vi "Plotter_Continuous_Receiver.vi"(8 "error in (no error)":errorcluster, 11 "Global Variables":T1) -> ()   [LabVIEW 2017]
uses:
  Controls/Plotter_Globals.ctl
  Classes/ADCP.lvclass
  Controls/Plotter_Queues.ctl
  Controls/Plotter_Queue_Command_and_Data.ctl
  Controls/Plotter_Commands.ctl
  <vilib>/Instr/_visa.llb/VISA Flush IO Buffer Mask.ctl
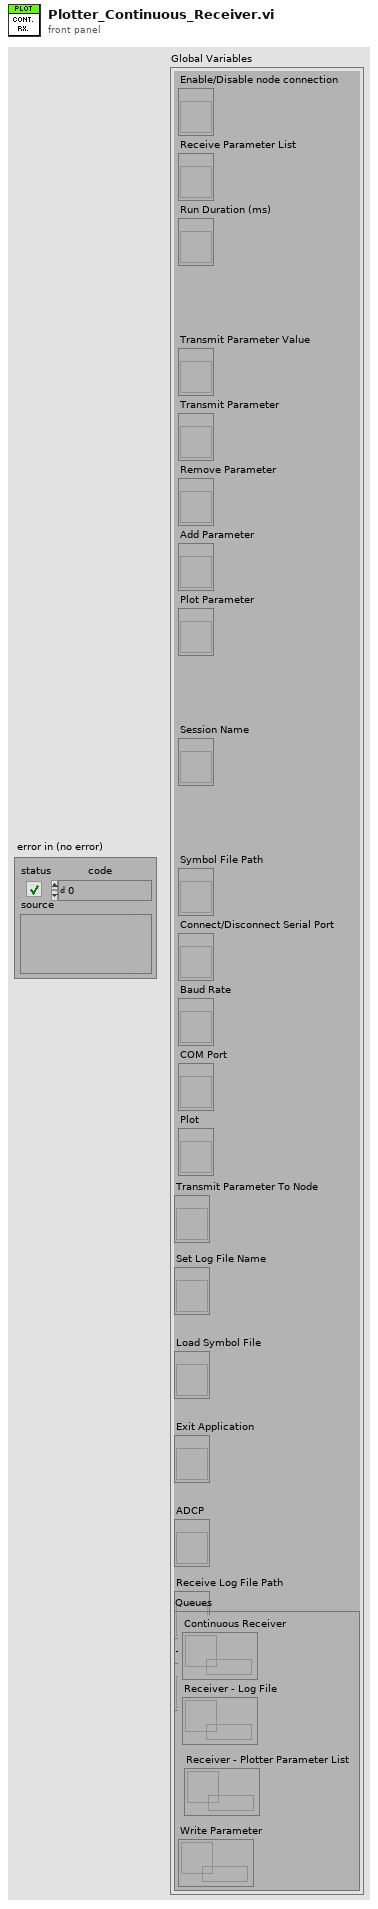
[diagram p1: front panel]
types:
  T1 = typedef "Plotter_Globals.ctl" = cluster{"Enable/Disable node connection":refnum<vi>, "Receive Parameter List":refnum<vi>, "Run Duration (ms)":refnum<vi>, "Transmit Parameter Value":refnum<vi>, "Transmit Parameter":refnum<vi>, "Remove Parameter":refnum<vi>, "Add Parameter":refnum<vi>, "Plot Parameter":refnum<vi>, "Session Name":refnum<vi>, "Symbol File Path":refnum<vi>, "Connect/Disconnect Serial Port":refnum<vi>, "Baud Rate":refnum<vi>, "COM Port":refnum<vi>, "Plot":refnum<vi>, "Transmit Parameter To Node":refnum<vi>, "Set Log File Name":refnum<vi>, "Load Symbol File":refnum<vi>, "Exit Application":refnum<vi>, "ADCP":refnum<vi>, "Transmit Log File Path":refnum<vi>, "Receive Log File Path":refnum<vi>, "Queues":T2}
  T2 = typedef "Plotter_Queues.ctl" = cluster{"Continuous Receiver":refnum<queue>, "Receiver - Log File":refnum<queue>, "Receiver - Plotter Parameter List":refnum<queue>, "Write Parameter":refnum<queue>}
  T3 = typedef "Plotter_Commands.ctl" = enum16{"Idle", "Cont_RX_Open_Node", "Cont_RX_Flush_Serial_Port", "Cont_Rx_Log_Write", "Plot_Update", "Exit"}
  T4 = typedef "Plotter_Queue_Command_and_Data.ctl" = cluster{"Commands":T3, "Data":variant}
  T5 = typedef "VISA Flush IO Buffer Mask.ctl" = u16
  T6 = typedef "ADCP.lvclass/ADCP_Packet_Info.ctl" = cluster{"Priority":enum16{"LOW", "HIGH"}, "Type":enum16{"Data", "Connection Management", "Remote Request", "Error and status", "INVALID"}, "Node ID":i32, "Frame ID":i32, "Checksum valid ?":bool, "Current time (ms)":u32}
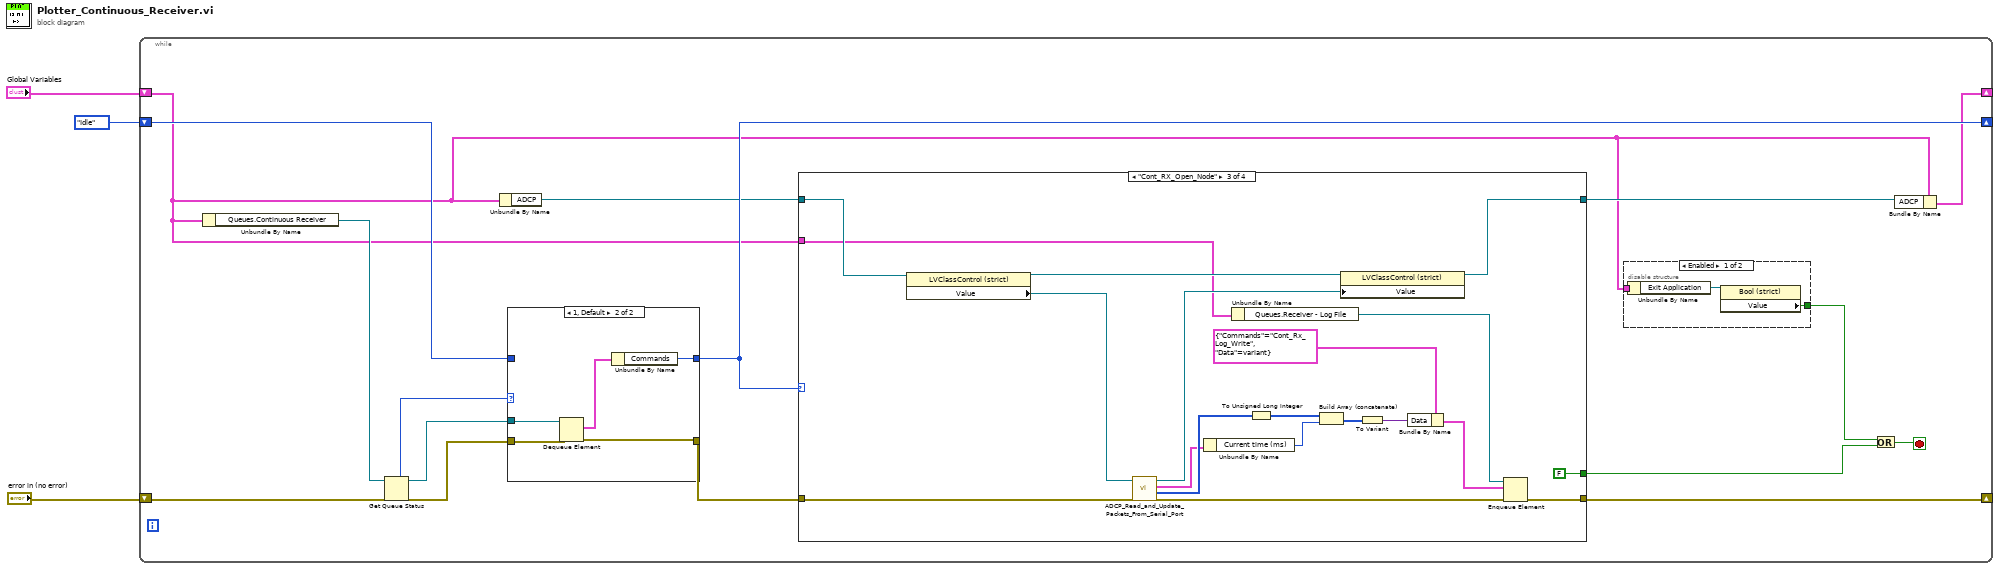
[diagram p0: block diagram]
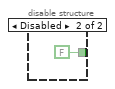
[diagram p2: hidden frame]
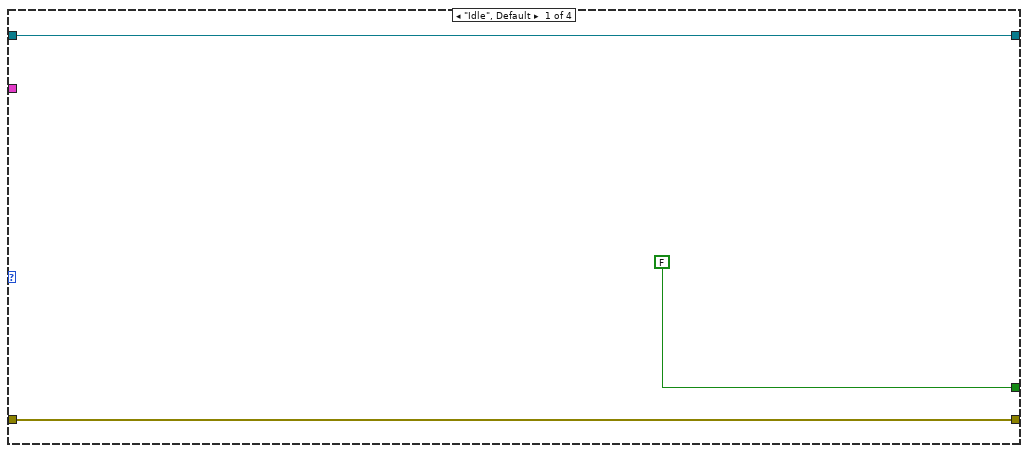
[diagram p3: hidden frame]
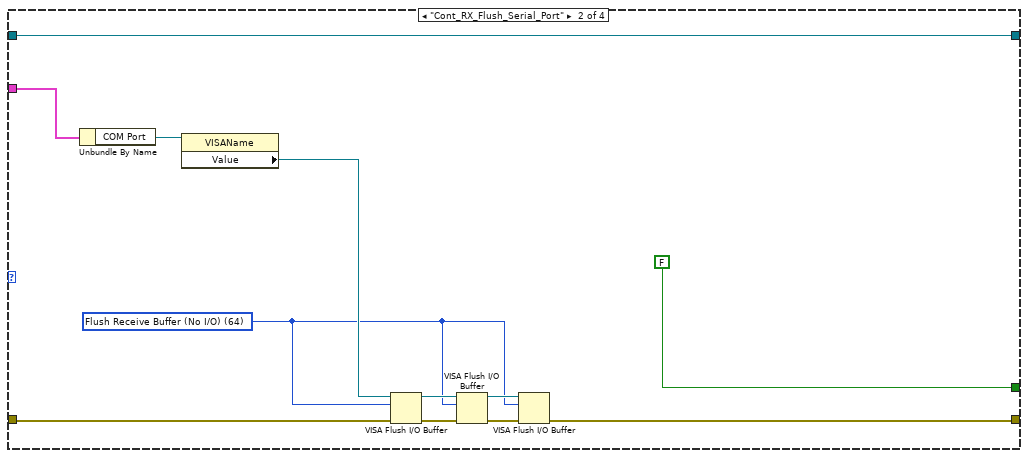
[diagram p4: hidden frame]
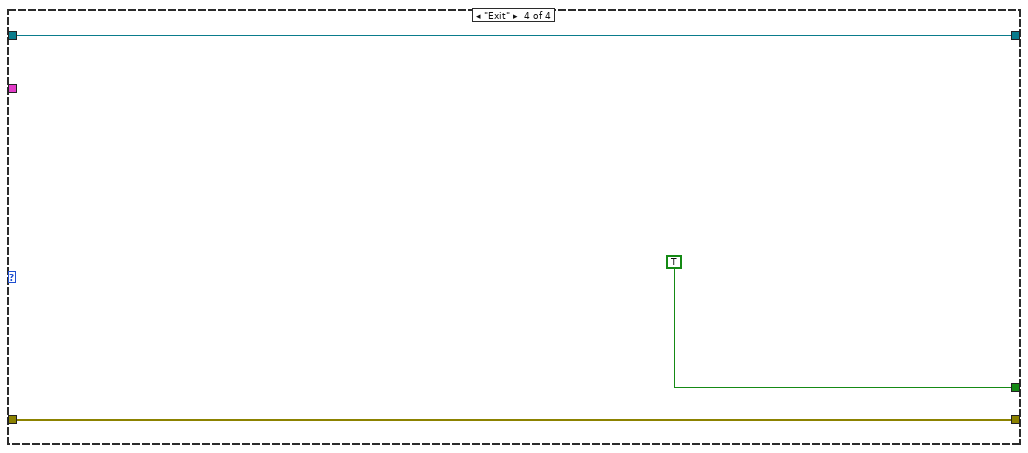
[diagram p5: hidden frame]
diagram:
  n1 = while {
    shift-right: [w11] -> _
    shift-left: "Global Variables" -> [w5]
    shift-right: [w14] -> _
    shift-left: Plotter_Commands."Idle" ("Commands") -> [w16]
    shift-right: [w13] -> _
    shift-left: "error in (no error)" -> [w12]
    stop <- w6 stop-if-true
    n2 = Unbundle By Name(w5) -> ("Queues.Continuous Receiver"=w19:refnum<queue>)
    n3 = Get Queue Status(queue=w19, error in (no error)=w12) -> (queue out=w8:refnum<queue>, error out=w18:errorcluster, # elements in queue=w17:i32)  [unwired: 1 in, 5 out]
    n4 = Unbundle By Name(w5) -> ("ADCP"=w10:refnum<vi>)
    n5 = case shown="1, Default" w17 {
      tunnel: w18 -> [w62 w67]
      tunnel: [w62 w66] -> w15
      tunnel: w8 -> [_ w65]
      tunnel: [w61 w63] -> w14
      tunnel: w16 -> [w61 _]
      frame 0 {
      }
      frame 1, Default {
        n6 = Dequeue Element(queue=w65, error in (no error)=w67) -> (element=w64:T4, error out=w66:errorcluster)  [unwired: 1 in, 2 out]
        n7 = Unbundle By Name(w64) -> ("Commands"=w63:T3)
      }
    }
    n8 = case shown="\"Cont_RX_Open_Node\"" w14 {
      tunnel: w15 -> [w26 w34 w56 w60]
      tunnel: [w26 w28 w48 w60] -> w13
      tunnel: [FALSE FALSE FALSE TRUE] -> w7
      tunnel: w10 -> [w24 w37 w55 w58]
      tunnel: [w24 w37 w51 w58] -> w9
      tunnel: w5 -> [_ w36 w50 _]
      frame "Idle", Default {
      }
      frame "Cont_RX_Flush_Serial_Port" {
        w27 = T5 64 items=["Flush Receive Buffer"=16, "Write Transmit Buffer to Device"=32, "Flush Receive Buffer (No I/O)"=64, "Flush Transmit Buffer"=128] ("Mask")
        n9 = Unbundle By Name(w36) -> ("COM Port"=w35:refnum<vi>)
        n10 = property class="VISAName"(reference=w35) -> ("Value"=w33:refnum<visa-resource-name>)  [unwired: 1 in, 2 out]
        n11 = VISA Flush I/O Buffer(VISA resource name=w33, mask (16)=w27, error in (no error)=w34) -> (VISA resource name out=w31:refnum<visa-resource-name>, error out=w32:errorcluster)
        n12 = VISA Flush I/O Buffer(VISA resource name=w31, mask (16)=w27, error in (no error)=w32) -> (VISA resource name out=w29:refnum<visa-resource-name>, error out=w30:errorcluster)
        n13 = VISA Flush I/O Buffer(VISA resource name=w29, mask (16)=w27, error in (no error)=w30) -> (error out=w28:errorcluster)  [unwired: 1 out]
      }
      frame "Cont_RX_Open_Node" {
        n14 = property class="LVClassControl (strict)"(reference=w55) -> (reference out=w53:refnum<vi>, "Value"=w54:refnum<class "ADCP.lvclass">)  [unwired: 1 in, 1 out]
        n15 = call "ADCP_Read_and_Update_Packets_From_Serial_Port.vi"("error in (no error)"=w56, "ADCP In"=w54) -> ("error out"=w49:errorcluster, "Received Packet"=w46:u8[], "Packet Info"=w44:T6, "ADCP out"=w52:refnum<class "ADCP.lvclass">)  [unwired: 6 in]
        n16 = Unbundle By Name(w44) -> ("Current time (ms)"=w43:u32)
        n17 = Unbundle By Name(w50) -> ("Queues.Receiver - Log File"=w47:refnum<queue>)
        n18 = To Unsigned Long Integer(number=w46) -> (unsigned 32bit integer=w45:u32[])
        n19 = Build Array (concatenate)(w45, w43) -> (w42:u32[])
        n20 = property class="LVClassControl (strict)"(reference=w53, "Value"=w52) -> (reference out=w51:refnum<vi>)  [unwired: 1 in, 1 out]
        n21 = To Variant(anything=w42) -> (Variant=w40:variant)
        n22 = Bundle By Name(cluster=T4 {"Commands"=enum."Cont_Rx_Log_Write", "Data"=variant} ("element"), "Data"=w40) -> (w39:T4)
        n23 = Enqueue Element(queue=w47, element=w39, error in (no error)=w49) -> (error out=w48:errorcluster)  [unwired: 1 in, 2 out]
      }
      frame "Exit" {
      }
    }
    n24 = disable-structure shown="Enabled" {
      disable-tunnel: w5 -> [w22 _]
      disable-tunnel: [w20 FALSE ("Value")] -> w4
      frame Enabled {
        n25 = Unbundle By Name(w22) -> ("Exit Application"=w21:refnum<vi>)
        n26 = property class="Bool (strict)"(reference=w21) -> ("Value"=w20:bool)  [unwired: 1 in, 2 out]
      }
      frame Disabled {
      }
    }
    n27 = Or(x=w4, y=w7) -> (x .or. y?=w6:bool)
    n28 = Bundle By Name(cluster=w5, "ADCP"=w9) -> (w11:T1)
  }
